vi "RoboRealm Vision Variable Processing.vi"(0 "connection ID in":refnum<k5>, 1 "Camera ID":string, 2 "Image Width":string, 3 "Image Height":string, 5 "UP IP Address":string, 11 "error in":errorcluster, 13 "remote port or service name":u16=1181) -> (4 "connection ID out":refnum<k5>, 6 "COG_BOX_SIZE":i32, 8 "COG X":i32, 10 "COG Y":i32, 12 "FPS":i32, 15 "error out":errorcluster)   [LabVIEW 2016]
panel:
  out "remaining string":string
  out "offset past scan":u32
  out "XY Blob Plot":cluster{"Y":dbl[], "Y":dbl[]}[](graph)
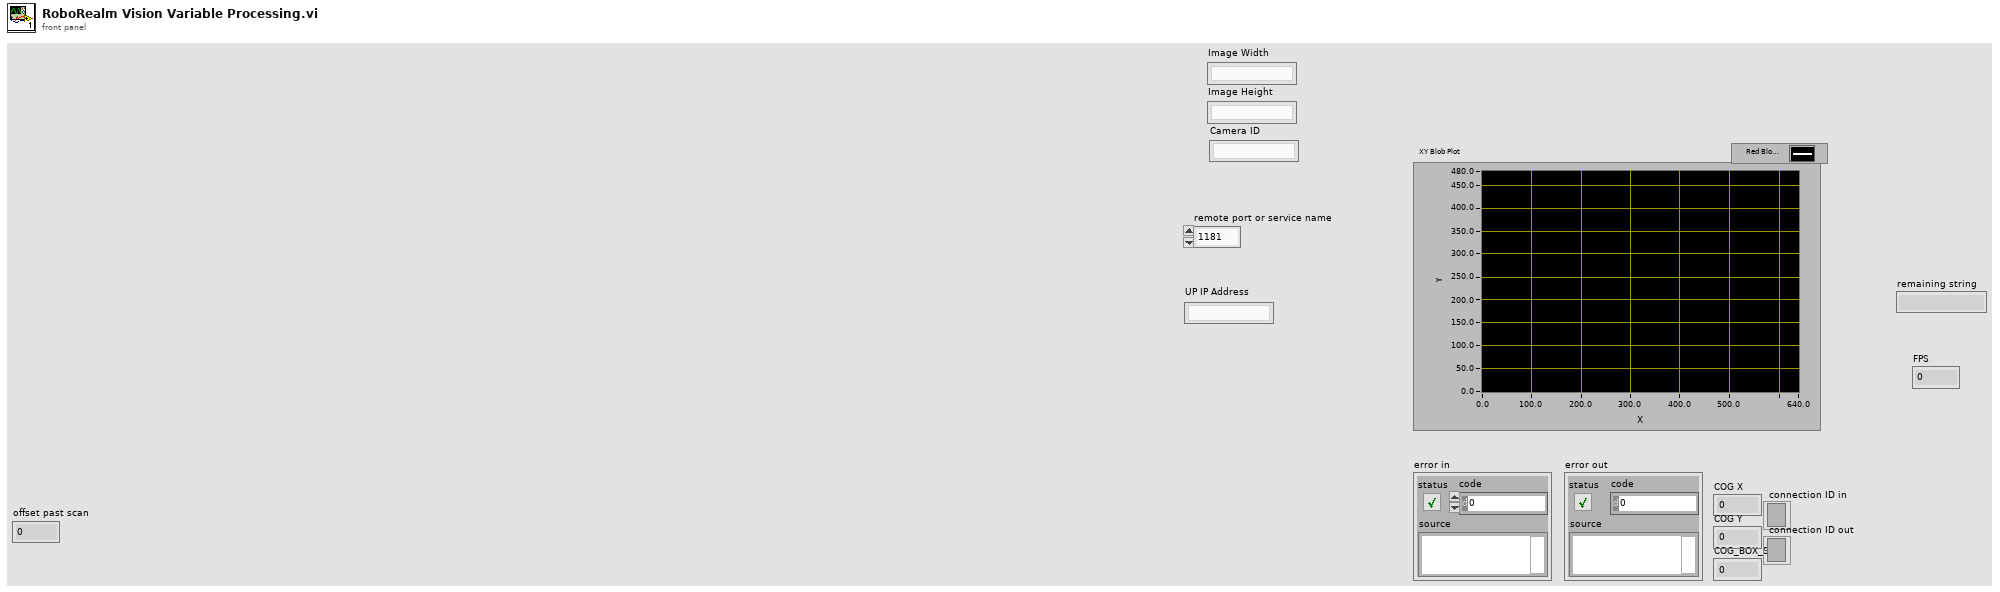
[diagram p1: front panel]
types:
  T1 = enum16{"Standard", "Buffered", "CRLF", "Immediate"}
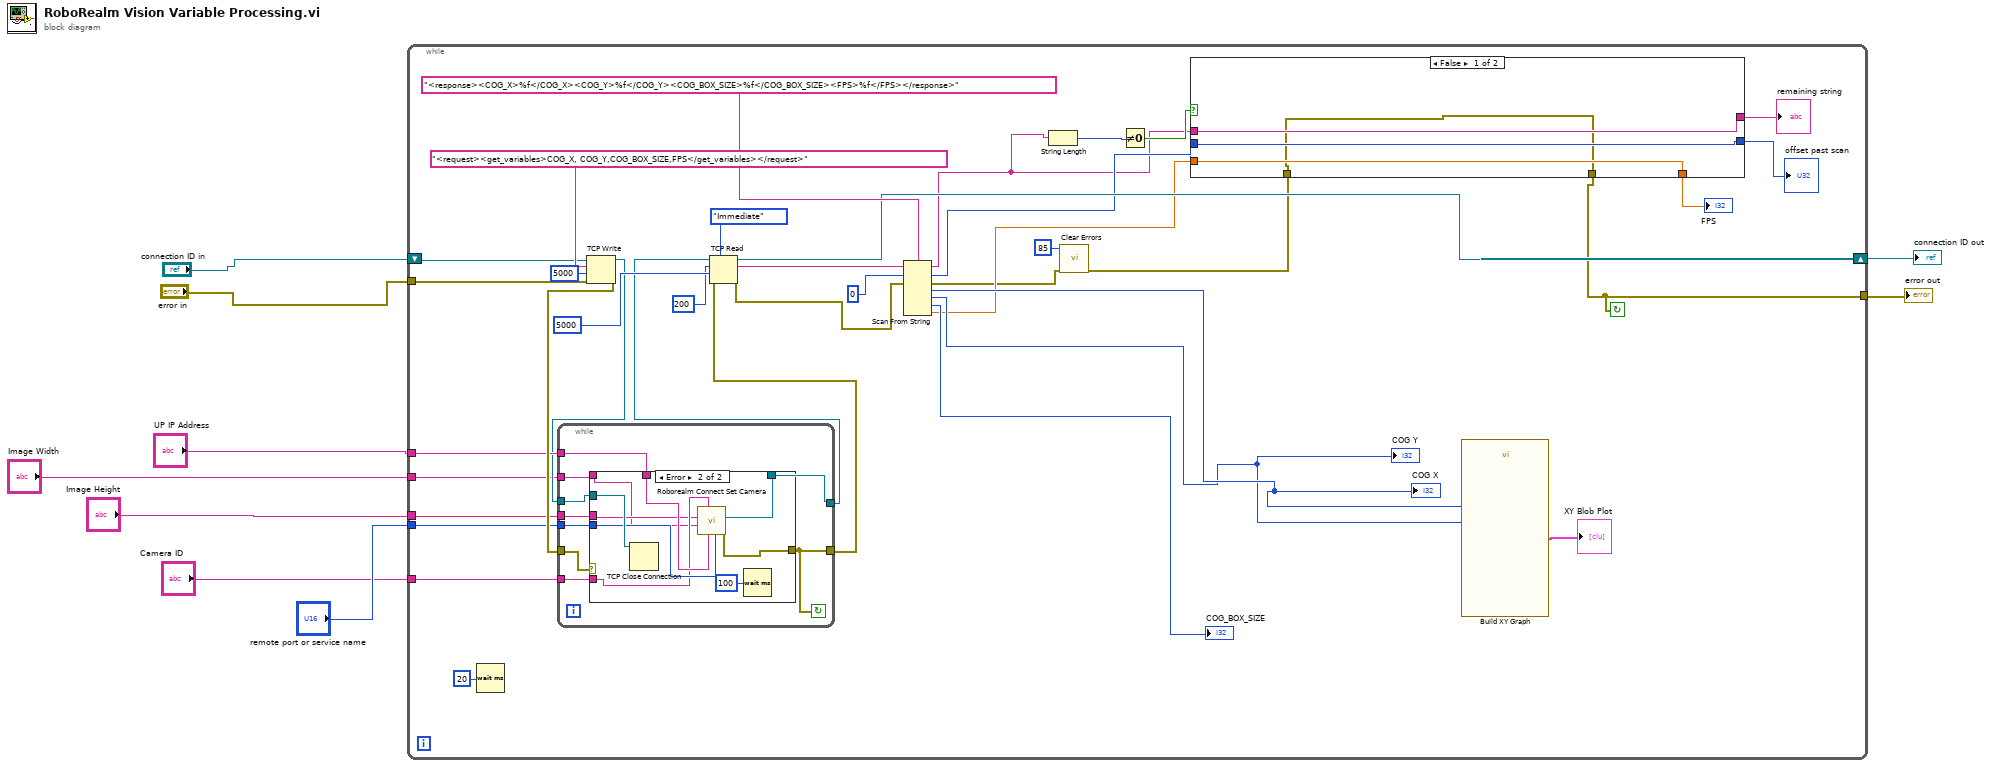
[diagram p0: block diagram]
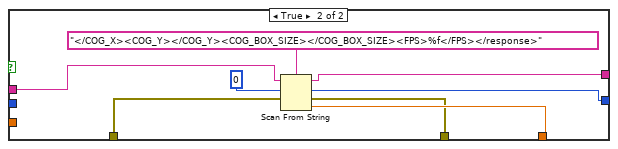
[diagram p2: hidden frame]
diagram:
  n1 = while {
    shift-right: [w29] -> w6
    shift-left: "connection ID in" -> [w39]
    tunnel: "UP IP Address" -> [w37]
    tunnel: "error in" -> [w38]
    tunnel: "remote port or service name" -> [w28]
    tunnel: [w14] -> w4
    tunnel: "Image Width" -> [w12]
    tunnel: "Image Height" -> [w11]
    tunnel: "Camera ID" -> [w10]
    stop <- w14 continue-if-true
    n2 = Wait (ms)(milliseconds to wait=u32 20) -> ()  [unwired: 1 out]
    n3 = TCP Write(connection ID=w39, data in="<request><get_variables>COG_X, COG_Y,COG_BOX_SIZE,FPS</get_variables></request>", error in (no error)=w38, 9:5000 ("timeout ms (25000)")) -> (connection ID out=w36:refnum<k5>, error out=w40:errorcluster)  [unwired: 1 out]
    n4 = while {
      tunnel: w37 -> [w66]
      tunnel: [w65] -> w35
      tunnel: w36 -> [w64]
      tunnel: w40 -> [w68]
      tunnel: [w67] -> w20
      tunnel: w28 -> [w63]
      tunnel: w12 -> [w62]
      tunnel: w11 -> [w61]
      tunnel: w10 -> [w60]
      stop <- w67 continue-if-true
      n5 = case shown="Error" w68 {
        selector: w68 -> [w70 _]
        tunnel: [w70 w76] -> w67
        tunnel: [w69 w77] -> w65
        tunnel: w64 -> [w69 w78]
        tunnel: w66 -> [_ w74]
        tunnel: w63 -> [_ w75]
        tunnel: w62 -> [_ w71]
        tunnel: w61 -> [_ w72]
        tunnel: w60 -> [_ w73]
        frame No Error {
        }
        frame Error {
          n6 = TCP Close Connection(connection ID=w78) -> ()  [unwired: 2 in, 2 out]
          n7 = call "Roborealm Connect Set Camera.vi"("remote port or service name"=w75, "UP IP Address"=w74, "Camera"=w73, "Width"=w71, "Height"=w72) -> ("error out"=w76:errorcluster, "connection ID out"=w77:refnum<k5>)  [unwired: 5 in]
          n8 = Wait (ms)(milliseconds to wait=u32 100) -> ()  [unwired: 1 out]
        }
      }
    }
    n9 = TCP Read(connection ID=w35, bytes to read=200, error in (no error)=w20, 7:T1."Immediate" ("mode (standard)"), 9:5000 ("bytes to read")) -> (connection ID out=w29:refnum<k5>, data out=w41:string, error out=w15:errorcluster)
    n10 = Scan From String(format string="<response><COG_X>%f</COG_X><COG_Y>%f</COG_Y><COG_BOX_SIZE>%f</COG_BOX_SIZE><FPS>%f</FPS></response>", input string=w41, initial scan location=u32 0, error in=w15) -> (remaining string=w19:string, offset past scan=w25:u32, error out=w17:errorcluster, output 1=w32:i32, output 2=w30:i32, output 3=→"COG_BOX_SIZE":i32, output 4=w21:dbl)  [unwired: 4 in]
    "COG X" <- w32
    "COG Y" <- w30
    n11 = String Length(string=w19) -> (length=w18:i32)
    n12 = call <vilib>:"Clear Errors.vi"("error in (no error)"=w17, "specific error code to clear (0: all)"=85) -> ("error out"=w16:errorcluster)  [unwired: 4 in, 1 out]
    n13 = Not Equal To 0?(x=w18) -> (x != 0?=w26:bool)
    n14 = case shown="False" w26 {
      tunnel: w19 -> [w51 w57]
      tunnel: w25 -> [w50 _]
      tunnel: [w51 w56] -> w24
      tunnel: [w50 w55] -> w23
      tunnel: [w49 w54] -> w22
      tunnel: w21 -> [w49 _]
      tunnel: w16 -> [w48 w53]
      tunnel: [w48 w52] -> w14
      frame False {
      }
      frame True {
        n15 = Scan From String(format string="</COG_X><COG_Y></COG_Y><COG_BOX_SIZE></COG_BOX_SIZE><FPS>%f</FPS></response>", input string=w57, initial scan location=u32 0, error in=w53) -> (remaining string=w56:string, offset past scan=w55:u32, error out=w52:errorcluster, output 1=w54:dbl)  [unwired: 1 in]
      }
    }
    "offset past scan" <- w23
    "remaining string" <- w24
    "FPS" <- w22
    n16 = call "Build XY Graph"("Y Input"=w30, "X Input"=w32) -> ("XY Graph"=→"XY Blob Plot":cluster{"Y":dbl[], "Y":dbl[]}[])  [unwired: 8 in, 1 out]
  }
  "connection ID out" <- w6
  "error out" <- w4
